vi "Process Loop.vi"(11 "AppLogger in":refnum<class "AppLogger.lvclass">) -> (3 "AppLogger out":refnum<class "AppLogger.lvclass">)   [LabVIEW 2014, in "AppLogger.lvclass"]
uses:
  AppLogger.lvclass
  Class.Messenger/Messenger.lvclass
  <vilib>/GPower/VIRegister/VIRegister.lvlib
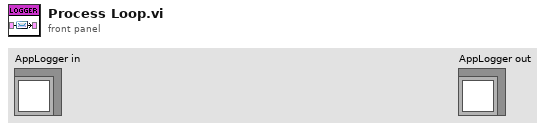
[diagram p1: front panel]
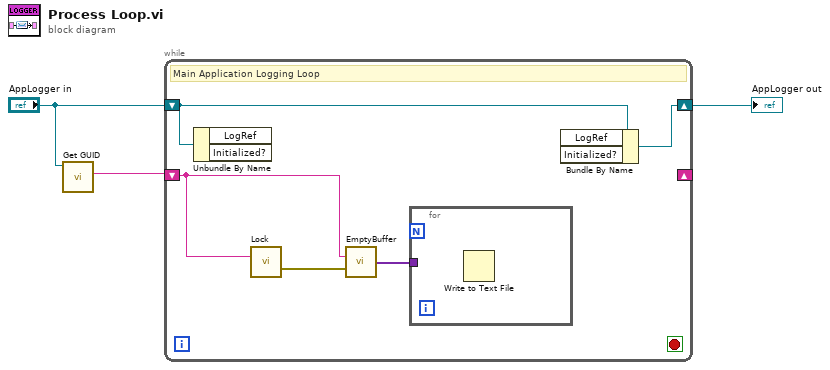
[diagram p0: block diagram]
diagram:
  n1 = call "Get GUID.vi"("Messenger in"="AppLogger in") -> ("GUID"=w2:string)  [unwired: 9 in, 1 out]
  n2 = while {
    shift-right: [w7] -> w3
    shift-left: "AppLogger in" -> [w8]
    shift-right: _ -> [_]
    shift-left: w2 -> [w6]
    stop <- _ stop-if-true
    # "Main Application Logging Loop"
    n3 = Unbundle By Name(w8) -> ()  [unwired: 2 out]
    n4 = call <vilib>:"Lock.vi"("Register name"=w6) -> ("Error out"=w5:errorcluster)  [unwired: 12 in, 2 out]
    n5 = call <vilib>:"EmptyBuffer.vi"("Register name"=w6, "Error in"=w5) -> ("Flushed buffer elements"=w4:variant[])  [unwired: 11 in, 2 out]
    n6 = for {
      tunnel: w4 -> [_]
      n7 = Write to Text File() -> ()  [unwired: 4 in, 3 out]
    }
    n8 = Bundle By Name(cluster=w8) -> (w7:refnum<class "AppLogger.lvclass">)  [unwired: 2 in]
  }
  "AppLogger out" <- w3
